vi "temperature_control_1.5.vi"(11 "User":string) -> ()   [LabVIEW 2014]
panel:
  in  "选项卡控件":T1(tab)
  in  "VISA resource name":refnum<visa-resource-name>="COM8" caption="VISA资源名称"
  in  "baud rate (9600)":u32=9600 caption="波特率(9600)"
  in  "data bits (8)":u16=8 caption="数据比特(8)" min=5 max=8 step=1
  in  "parity (0:none)":enum16{"None", "Odd", "Even", "Mark", "Space"}(ring) caption="奇偶（0:无）"
  in  "stop bits (10: 1 bit)":u16(ring)=10 caption="停止位（10: 1位）" items=["1.0"=10, "1.5"=15, "2.0"=20]
  in  "flow control (0:none)":u16(ring) caption="流控制（0:无）" items=["无", "XON/XOFF", "RTS/CTS", "XON/XOFF & RTS/CTS", "DTR/DSR", "XON/XOFF & DTR/DSR"]
  out "Console":string
  out "XY Graph":cluster{"Y":dbl[], "Y":dbl[]}[](graph) caption="XY图"
  out "Hello":string
  in  "Initialization confirm":bool
  in  "Reset":bool
  out "Working Status":string
  in  "电源开关":bool
  in  "变温控制":bool
  in  "停止":bool
  out "变温":bool
  in  "Desitination Value":dbl
  out "Expectation Value":dbl
  out "add_step":dbl=0.008
  in  "变温等待间隙":dbl=1.5 format="%.2f"
  out "电流设置回读":string
  out "电压值回读":string
  out "电压设置回读":string
  out "电流值回读":string
  out "过压设置值回读":string
  out "键盘锁":string="CC"
  out "过压":string="CC"
  out "蜂鸣器":string="CC"
  out "CC/CV":string="CC"
  out "测量模式":string="CC"
  out "过温":string="CC"
  out "On/Off":string="CC"
  out "日期/时间字符串":string
  in  "I-t_data":path
  out "数字":u32
  in  "log":path=path "E:/"
  in  "SET COMMAND":u16(ring) items=["CURRENT SET", "VOLTAGE SET", "ON/OFF", "LOCK SET", "OVPROTECT SET", "SOUND", ""]
  in  "数值":dbl
  in  "SET":bool
  out "RESULT":string
  in  "Read COMMAND":u16(ring) items=["CURRENT SET", "VOLTAGE SET", "ON/OFF", "LOCK SET", "OVPROTECT SET", "SOUND", ""]
  in  "Read":bool
  out "Value":string
  out "log":refnum<file>
  out "I-t data":refnum<file>
  in  "Turning Point4":dbl=4.0
  in  "Turing Pont3":dbl=3.5
  in  "Turning Point2":dbl=2.5
  in  "Turning Point1":dbl=1.5
  in  "step1":dbl=0.01
  in  "step2":dbl=0.008
  in  "step3":dbl=0.006
  in  "step4":dbl=0.005
  in  "step5":dbl=0.004
  in  "精度":dbl=0.01
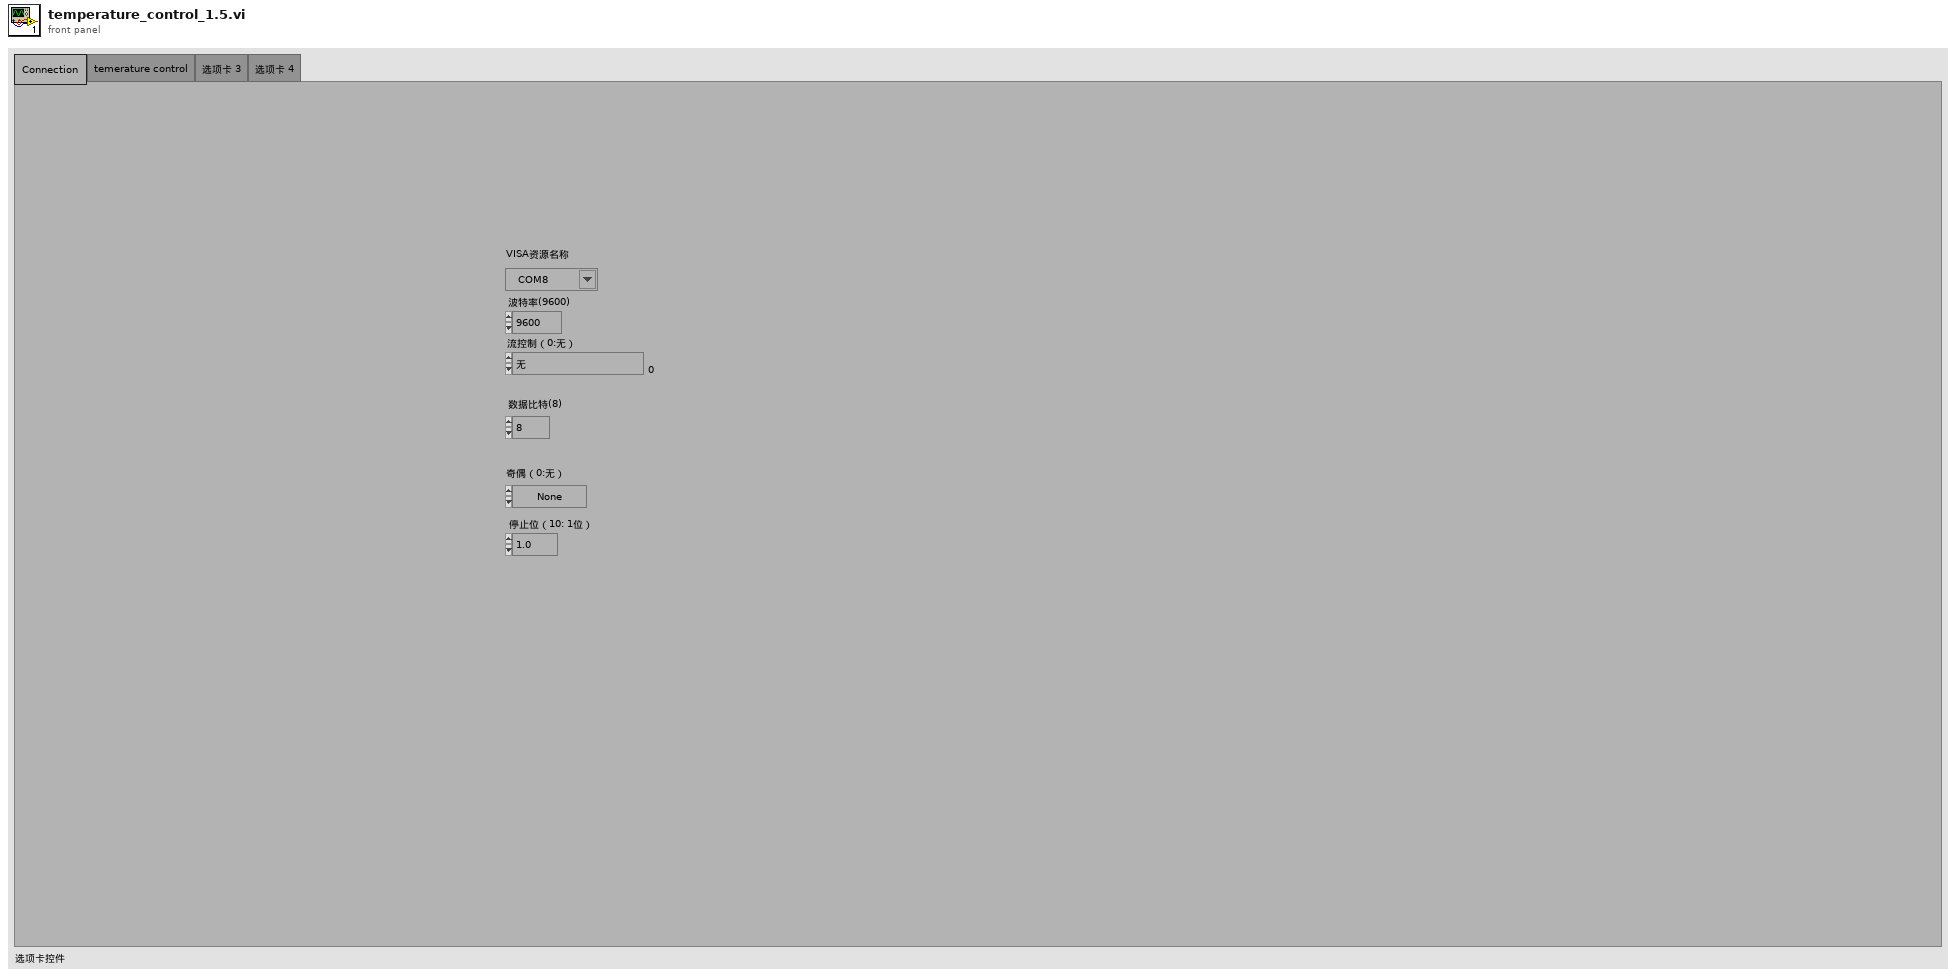
[diagram p1: front panel]
types:
  T1 = enum32{"Connection ", "temerature control", "选项卡 3", "选项卡 4"}
  T2 = enum16{"open", "replace", "create", "open or create", "replace or create", "replace or create with confirmation"}
  T3 = enum8{"Enabled", "Disabled", "Disabled and Grayed Out"}
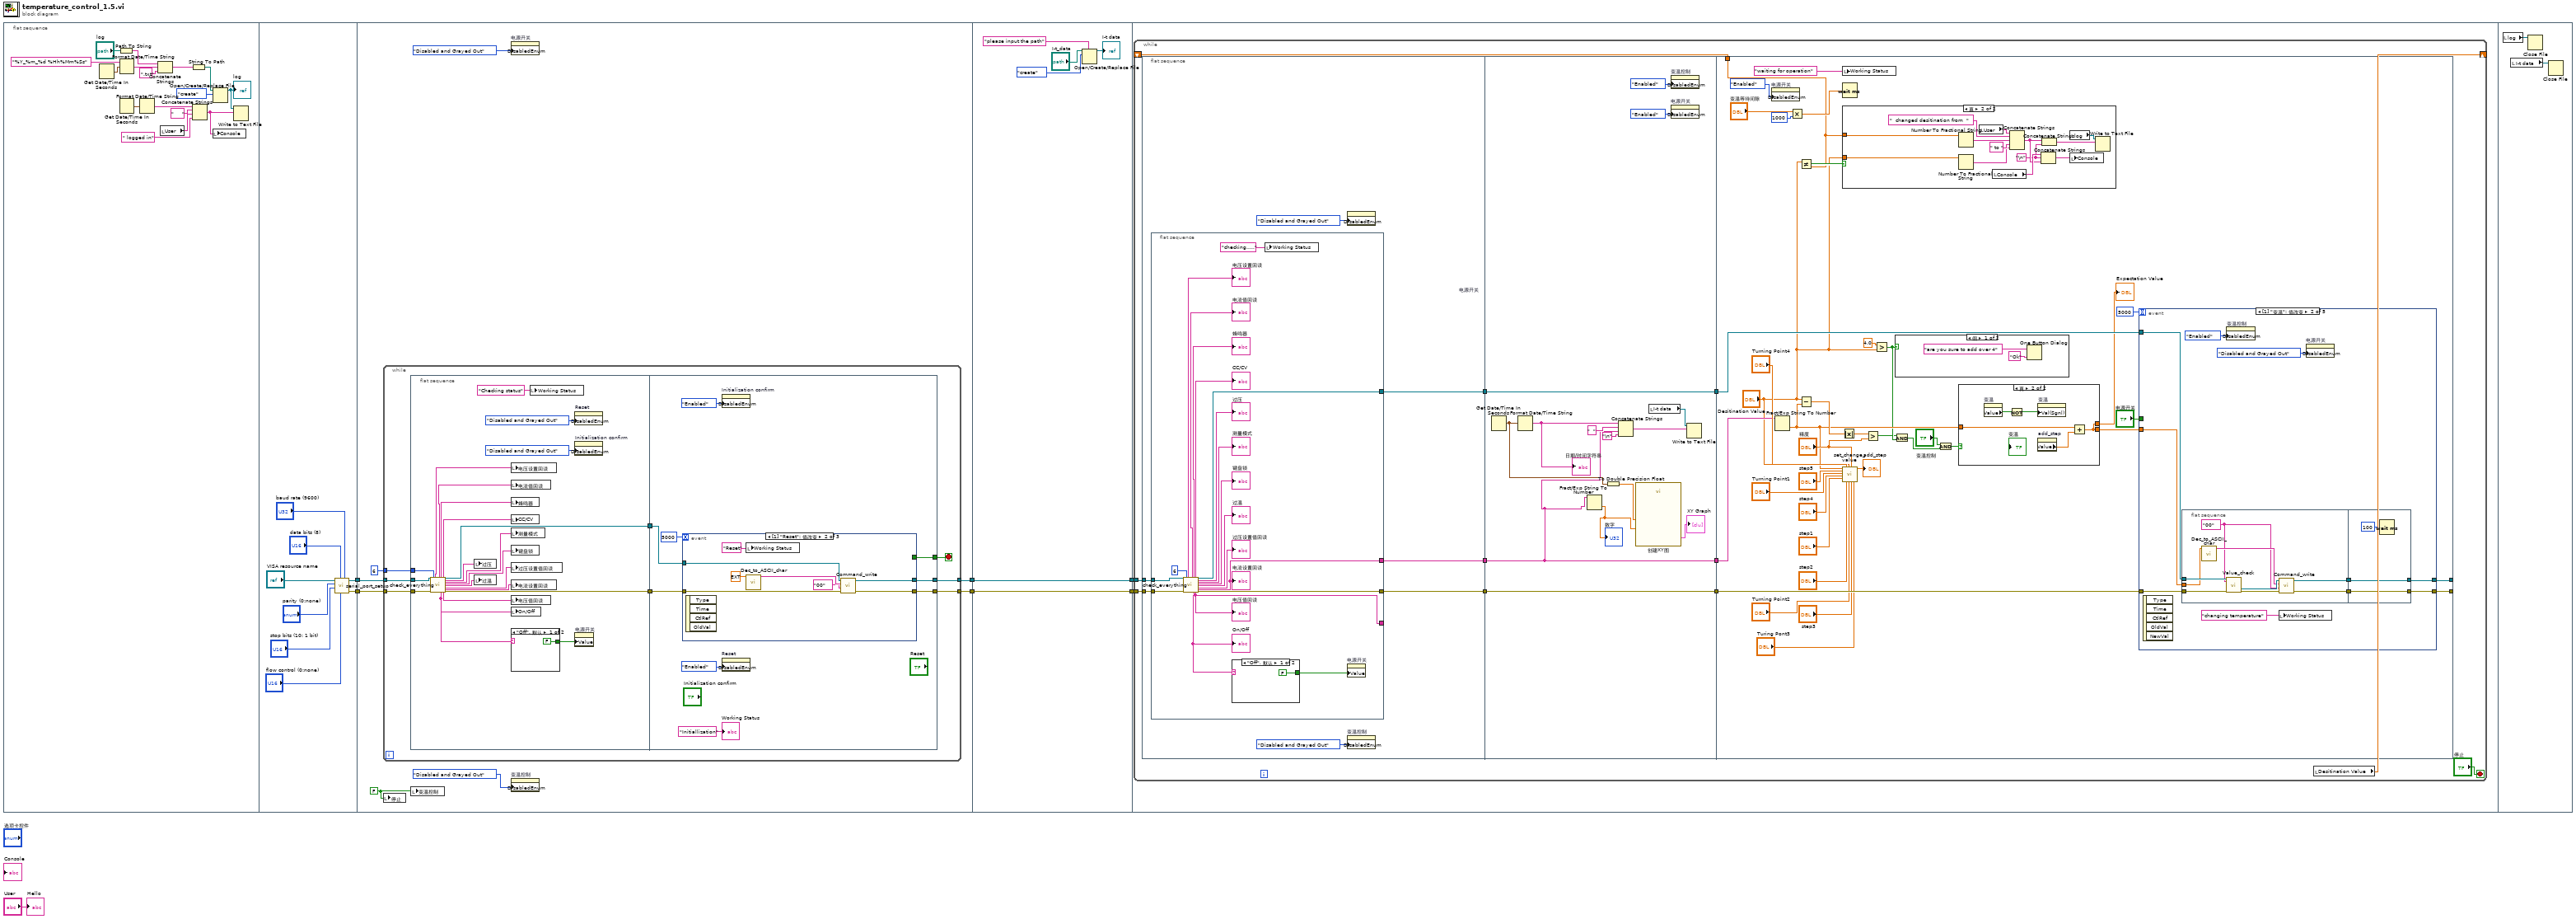
[diagram p0: block diagram]
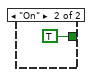
[diagram p2: hidden frame]
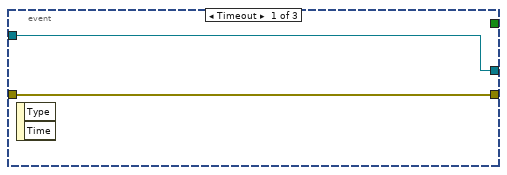
[diagram p3: hidden frame]
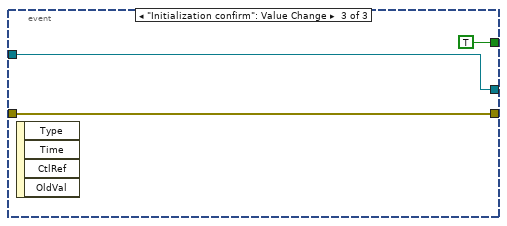
[diagram p4: hidden frame]
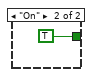
[diagram p5: hidden frame]
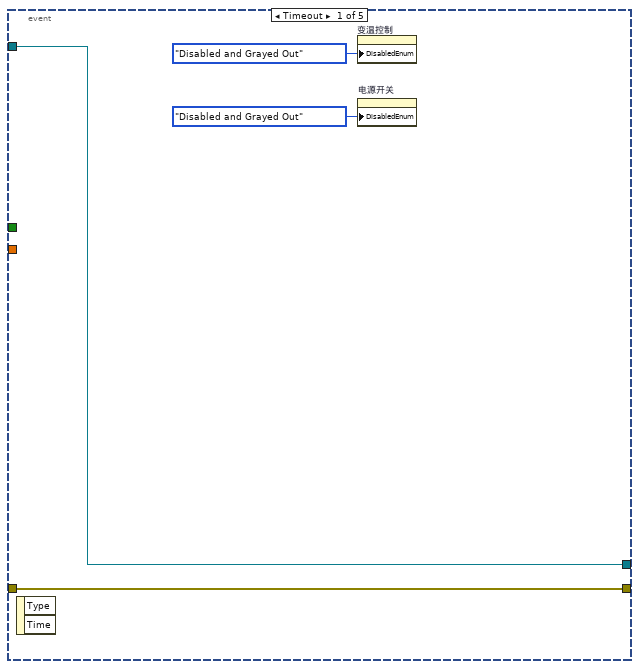
[diagram p9: hidden frame]
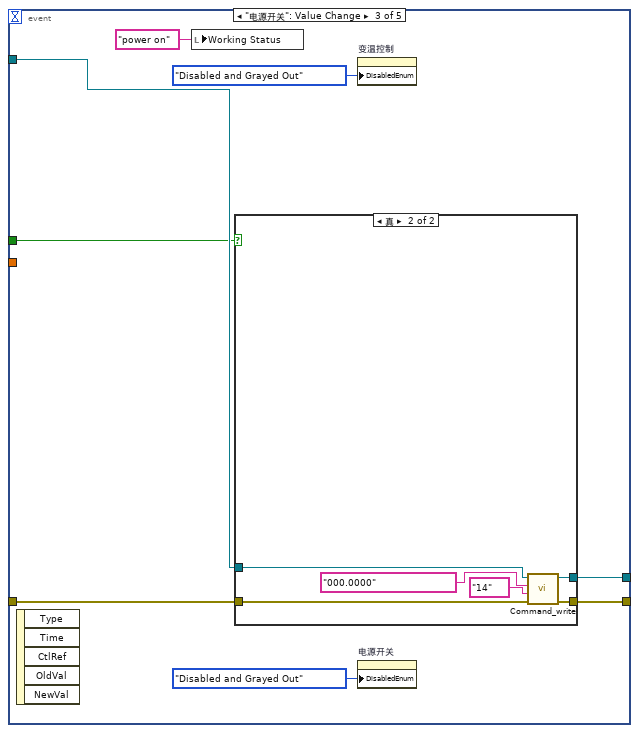
[diagram p10: hidden frame]
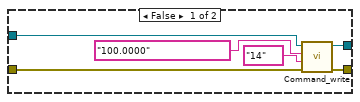
[diagram p11: hidden frame]
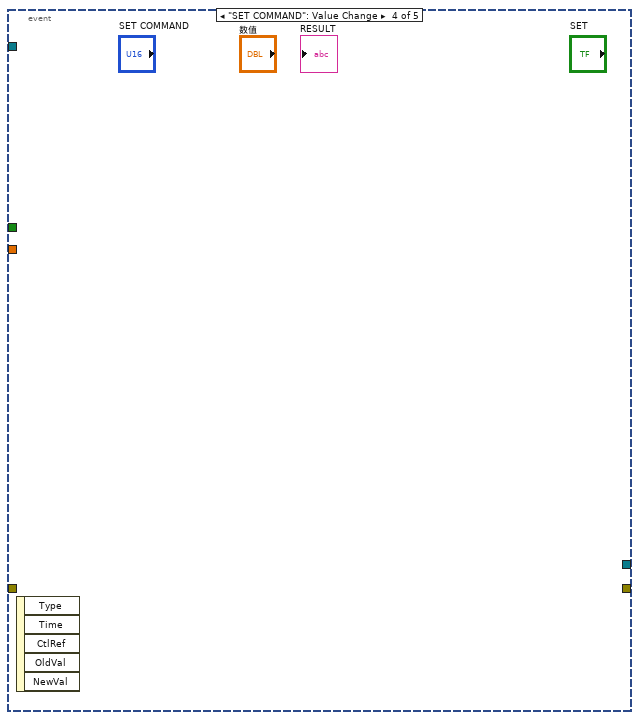
[diagram p12: hidden frame]
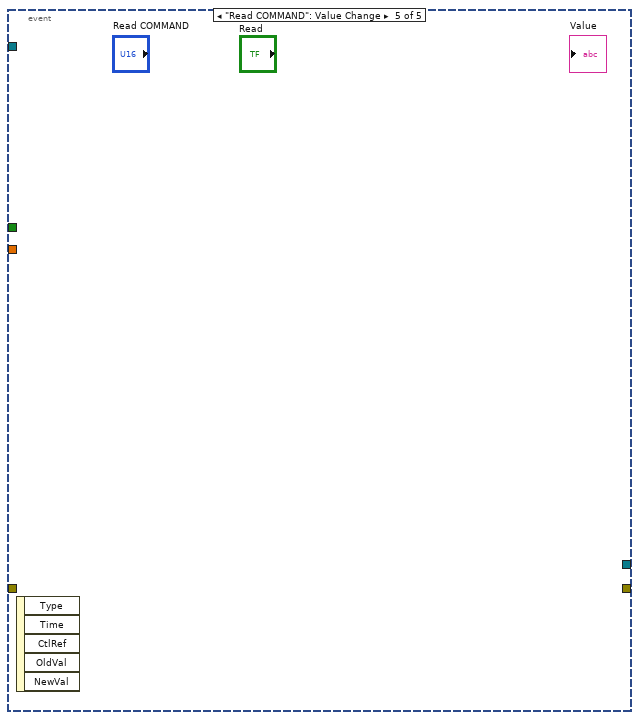
[diagram p13: hidden frame]
diagram:
  n1 = flat-sequence {
    tunnel: [w25] -> w7
    tunnel: [w24] -> w6
    tunnel: [w34] -> w4
    tunnel: w7 -> [w38]
    tunnel: w6 -> [w37]
    tunnel: [w33] -> w2
    tunnel: w4 -> [w98]
    tunnel: [w98] -> w3
    tunnel: w2 -> [w97]
    tunnel: [w97] -> w1
    tunnel: w3 -> [w100]
    tunnel: w1 -> [w99]
    frame #0 {
      n2 = Get Date/Time In Seconds() -> (seconds since 1Jan1904=w12:timestamp)
      n3 = Path To String(path="log") -> (string=w11:string)
      n4 = Format Date/Time String(time format string (%c)="%Y_%m_%d %Hh%Mm%Ss" ("时间格式字符串(%c)"), seconds (now)=w12) -> (date/time string=w17:string)  [unwired: 1 in]
      n5 = Get Date/Time In Seconds() -> (seconds since 1Jan1904=w22:timestamp)
      n6 = Format Date/Time String(seconds (now)=w22) -> (date/time string=w20:string)  [unwired: 2 in]
      n7 = Concatenate Strings(w11, w17, ".txt" ("字符串")) -> (w14:string)
      n8 = local read "User"() -> (w21:string)
      n9 = String To Path(string=w14) -> (path=w15:path)
      n10 = Concatenate Strings(w20, "     " ("字符串"), w21, " logged in" ("Console")) -> (w8:string)
      n11 = Open/Create/Replace File(file path (use dialog)=w15, operation (0:open)=T2."create" ("操作(0:open)")) -> (refnum out=w9:refnum<file>)  [unwired: 4 in, 2 out]
      "log" <- w9
      n12 = local write "Console"(w8) -> ()
      n13 = Write to Text File(file (use dialog)=w9, text=w8) -> ()  [unwired: 2 in, 3 out]
    }
    frame #1 {
      n14 = call "serial_port_setup.vi"("baud rate (9600)"="baud rate (9600)", "flow control (0:none)"="flow control (0:none)", "data bits (8)"="data bits (8)", "stop bits (10: 1 bit)"="stop bits (10: 1 bit)", "parity (0:none)"="parity (0:none)", "VISA引用句柄输入"="VISA resource name") -> ("错误输出"=w24:errorcluster, "VISA引用句柄输出"=w25:refnum<visa-resource-name>)  [unwired: 4 in]
    }
    frame #2 {
      w32 = FALSE ("停止")
      n15 = while {
        tunnel: 6 -> [w47]
        tunnel: w38 -> [w46]
        tunnel: w37 -> [w45]
        tunnel: [w41] -> w34
        tunnel: [w40] -> w33
        stop <- w42 stop-if-true
        n16 = flat-sequence {
          tunnel: w47 -> [w68]
          tunnel: w46 -> [w67]
          tunnel: w45 -> [w66]
          tunnel: [w65] -> w44
          tunnel: [w49] -> w43
          tunnel: w44 -> [w78]
          tunnel: w43 -> [w77]
          tunnel: [w76] -> w42
          tunnel: [w75] -> w41
          tunnel: [w74] -> w40
          frame #0 {
            n17 = call "check_everything.vi"("VISA引用句柄输入"=w67, "错误输入（无错误）"=w66, "数值输入"=w68) -> ("电压设置回读"=w62:string, "电流值回读"=w61:string, "蜂鸣器"=w54:string, "On/Off"=w51:string, "CC/CV"=w60:string, "电压值回读"=w57:string, "VISA引用句柄输出"=w65:refnum<visa-resource-name>, "过压"=w55:string, "测量模式"=w59:string, "键盘锁"=w56:string, "过温"=w58:string, "过压设置值回读"=w53:string, "电流设置回读"=w52:string, "错误输出"=w49:errorcluster)  [unwired: 10 in, 1 out]
            n18 = local write "过压"(w55) -> ()
            n19 = local write "过温"(w58) -> ()
            n20 = local write "电压设置回读"(w62) -> ()
            n21 = local write "电流值回读"(w61) -> ()
            n22 = local write "蜂鸣器"(w54) -> ()
            n23 = local write "CC/CV"(w60) -> ()
            n24 = local write "测量模式"(w59) -> ()
            n25 = local write "键盘锁"(w56) -> ()
            n26 = local write "过压设置值回读"(w53) -> ()
            n27 = local write "电流设置回读"(w52) -> ()
            n28 = local write "电压值回读"(w57) -> ()
            n29 = local write "On/Off"(w51) -> ()
            n30 = case shown="\"Off\", 默认" w51 {
              tunnel: [FALSE TRUE] -> w50
              frame "Off", Default {
              }
              frame "On" {
              }
            }
            n31 = local write "Working Status"("Checking status") -> ()
            n32 = property on="Reset" class="Bool"("DisabledEnum"=T3."Disabled and Grayed Out" ("禁用")) -> ()  [unwired: 2 in, 2 out]
            n33 = property on="Initialization confirm" class="Bool"("DisabledEnum"=T3."Disabled and Grayed Out" ("禁用")) -> ()  [unwired: 2 in, 2 out]
            n34 = property on="电源开关" class="Bool (严格)"("Value"=w50) -> ()  [unwired: 2 in, 2 out]
          }
          frame #1 {
            n35 = event shown="[1] \"Reset\": 值改变" {
              selector: _ -> [_ _ _]
              dyn-events: _ -> [_ _ _]
              timeout: u32 5000 ("y") -> [_ _ _]
              tunnel: [w81 w87 w92] -> w75
              tunnel: w78 -> [w81 w89 w92]
              tunnel: w77 -> [w80 w88 w91]
              tunnel: [w80 w86 w91] -> w74
              tunnel: [_ _ TRUE] -> w76
              event Timeout {
                n36 = event-data() -> ()  [unwired: 1 in, 2 out]
              }
              event "Reset": Value Change {
                n37 = event-data() -> ()  [unwired: 1 in, 4 out]
                n38 = local write "Working Status"("Reset") -> ()
                n39 = call "Dec_to_ASCII_char.vi"("SetPoint"=ext 0.0) -> ("字符串"=w85:string)  [unwired: 10 in]
                n40 = call "Command_write.vi"("错误输入（无错误）"=w88, "Status code"="00", "Data"=w85, "VISA引用句柄输入"=w89) -> ("错误输出"=w86:errorcluster, "VISA引用句柄输出"=w87:refnum<visa-resource-name>)  [unwired: 5 in, 1 out]
              }
              event "Initialization confirm": Value Change {
                n41 = event-data() -> ()  [unwired: 1 in, 4 out]
              }
            }
            n42 = property on="Initialization confirm" class="Bool"("DisabledEnum"=T3."Enabled" ("禁用")) -> ()  [unwired: 2 in, 2 out]
            n43 = property on="Reset" class="Bool"("DisabledEnum"=T3."Enabled" ("禁用")) -> ()  [unwired: 2 in, 2 out]
            "Working Status" <- "Initiallization"
          }
        }
      }
      n44 = local write "停止"(w32) -> ()
      n45 = local write "变温控制"(w32) -> ()
      n46 = property on="电源开关" class="Bool (严格)"("DisabledEnum"=T3."Disabled and Grayed Out" ("禁用")) -> ()  [unwired: 2 in, 2 out]
      n47 = property on="变温控制" class="Bool (严格)"("DisabledEnum"=T3."Disabled and Grayed Out" ("禁用")) -> ()  [unwired: 2 in, 2 out]
    }
    frame #3 {
      n48 = Open/Create/Replace File(file path (use dialog)="I-t_data", prompt="please input the path" ("提示"), operation (0:open)=T2."create" ("操作(0:open)")) -> (refnum out=→"I-t data":refnum<file>)  [unwired: 3 in, 2 out]
    }
    frame #4 {
      n49 = while {
        tunnel: w100 -> [w111]
        tunnel: w99 -> [w110]
        shift-right: [w102] -> _
        shift-left: _ -> [w101]
        stop <- "停止" stop-if-true
        n50 = flat-sequence {
          tunnel: w110 -> [w117]
          tunnel: w111 -> [w118]
          tunnel: [w115] -> w108
          tunnel: [w116] -> w106
          tunnel: [w114] -> w104
          tunnel: w108 -> [w153]
          tunnel: [w153] -> w107
          tunnel: w106 -> [w140]
          tunnel: [w140] -> w105
          tunnel: w104 -> [w152]
          tunnel: [w152] -> w103
          tunnel: [w168] -> _
          tunnel: w107 -> [w189]
          tunnel: w105 -> [w167]
          tunnel: w103 -> [w188]
          tunnel: [w166] -> _
          tunnel: w101 -> [w155]
          frame #0 {
            n51 = flat-sequence {
              tunnel: w118 -> [w127]
              tunnel: w117 -> [w126]
              tunnel: [w125] -> w116
              tunnel: [w124] -> w115
              tunnel: [w123] -> w114
              tunnel: [w119] -> _
              frame #0 {
                n52 = call "check_everything.vi"("VISA引用句柄输入"=w127, "错误输入（无错误）"=w126, "数值输入"=6) -> ("电压设置回读"=→"电压设置回读":string, "电流值回读"=→"电流值回读":string, "蜂鸣器"=→"蜂鸣器":string, "On/Off"=w120:string, "CC/CV"=→"CC/CV":string, "电压值回读"=w119:string, "VISA引用句柄输出"=w124:refnum<visa-resource-name>, "过压"=→"过压":string, "测量模式"=→"测量模式":string, "键盘锁"=→"键盘锁":string, "过温"=→"过温":string, "过压设置值回读"=→"过压设置值回读":string, "电流设置回读"=w125:string, "错误输出"=w123:errorcluster)  [unwired: 10 in, 1 out]
                "On/Off" <- w120
                "电压值回读" <- w119
                "电流设置回读" <- w125
                n53 = case shown="\"Off\", 默认" w120 {
                  tunnel: [FALSE TRUE] -> w121
                  frame "Off", Default {
                  }
                  frame "On" {
                  }
                }
                n54 = local write "Working Status"("checking.....") -> ()
                n55 = property on="电源开关" class="Bool (严格)"("Value"=w121) -> ()  [unwired: 2 in, 2 out]
              }
            }
            n56 = property on="电源开关" class="Bool (严格)"("DisabledEnum"=T3."Disabled and Grayed Out" ("禁用")) -> ()  [unwired: 2 in, 2 out]
            n57 = property on="变温控制" class="Bool (严格)"("DisabledEnum"=T3."Disabled and Grayed Out" ("禁用")) -> ()  [unwired: 2 in, 2 out]
          }
          frame #1 {
            n58 = Get Date/Time In Seconds() -> (seconds since 1Jan1904=w144:timestamp)
            n59 = Format Date/Time String(seconds (now)=w144) -> (date/time string=w145:string)  [unwired: 2 in]
            "日期/时间字符串" <- w145
            n60 = Fract/Exp String To Number(string=w140) -> (number=w141:dbl)  [unwired: 3 in, 1 out]
            "数字" <- w141
            n61 = To Double Precision Float(number=w144) -> (double precision float=w143:dbl)
            n62 = Concatenate Strings(w145, "  " ("字符串"), w140, "\n") -> (w146:string)
            n63 = call "创建XY图"("Y Input"=w141, "X Input"=w143) -> ("XY Graph"=→"XY Graph":cluster{"X":dbl[], "Y":dbl[]}[])  [unwired: 8 in, 1 out]
            n64 = local read "I-t data"() -> (w147:refnum<file>)
            n65 = property on="变温控制" class="Bool (严格)"("DisabledEnum"=T3."Enabled" ("禁用")) -> ()  [unwired: 2 in, 2 out]
            n66 = property on="电源开关" class="Bool (严格)"("DisabledEnum"=T3."Enabled" ("禁用")) -> ()  [unwired: 2 in, 2 out]
            n67 = Write to Text File(file (use dialog)=w147, text=w146) -> ()  [unwired: 2 in, 3 out]
          }
          frame #2 {
            n68 = property on="电源开关" class="Bool (严格)"("DisabledEnum"=T3."Enabled" ("禁用")) -> ()  [unwired: 2 in, 2 out]
            n69 = Fract/Exp String To Number(string=w167) -> (number=w170:dbl)  [unwired: 3 in, 1 out]
            n70 = Multiply(x="变温等待间隙", y=u32 1000) -> (x*y=w164:dbl)
            n71 = Not Equal?(x="Desitination Value", y=w155) -> (x != y?=w156:bool)
            n72 = Subtract(x="Desitination Value", y=w170) -> (x-y=w184:dbl)
            n73 = Absolute Value(x=w184) -> (abs(x)=w183:dbl)
            n74 = local write "Working Status"("waiting for operation") -> ()
            n75 = Wait (ms)(milliseconds to wait=w164) -> ()  [unwired: 1 out]
            n76 = case shown="真" w156 {
              tunnel: w155 -> [_ w194]
              tunnel: "Desitination Value" -> [_ w192]
              frame False {
              }
              frame True {
                w195 = "\n"
                n77 = Number To Fractional String(number=w194) -> (F-format string=w193:string)  [unwired: 3 in]
                n78 = Number To Fractional String(number=w192) -> (F-format string=w191:string)  [unwired: 3 in]
                n79 = local read "User"() -> (w201:string)
                n80 = local read "Console"() -> (w199:string)
                n81 = Concatenate Strings(w201, "  changed desitination from  ", w193, " to " ("字符串"), w191) -> (w196:string)
                n82 = Concatenate Strings(w199, w195, w196) -> (w198:string)
                n83 = Concatenate Strings(w196, w195) -> (w197:string)
                n84 = local read "log"() -> (w203:refnum<file>)
                n85 = local write "Console"(w198) -> ()
                n86 = Write to Text File(file (use dialog)=w203, text=w197) -> ()  [unwired: 2 in, 3 out]
              }
            }
            n87 = call "set_change_value.vi"("数值输入"=w170, "step5"="step5", "Turning Point1"="Turning Point1", "step4"="step4", "step1"="step1", "Turning Point4"="Turning Point4", "step2"="step2", "Desitination Value"="Desitination Value", "Turning Point2"="Turning Point2", "精度"="精度", "step3"="step3", "Turing Pont3"="Turing Pont3") -> ("数值输出"=→"add_step":sgl)  [unwired: 7 in]
            n88 = Greater?(x=w183, y="精度") -> (0:w158:bool)
            n89 = Greater?(x=4.0, y="Desitination Value") -> (0:w159:bool)
            n90 = And(x=w158, y=w159) -> (x .and. y?=w157:bool)
            n91 = case shown="假" w159 {
              frame False {
                n92 = One Button Dialog(message="are you sure to add over 4", button name ("OK")="Ok") -> ()  [unwired: 1 out]
              }
              frame True {
              }
            }
            n93 = And(x="变温控制", y=w157) -> (x .and. y?=w187:bool)
            n94 = case shown="真" w187 {
              tunnel: w170 -> [w206 w209]
              tunnel: [w206 w207] -> w185
              tunnel: [w206 w207] -> w181
              frame False {
              }
              frame True {
                n95 = property on="变温" class="Bool (严格)"() -> ("Value"=w211:bool)  [unwired: 2 in, 2 out]
                n96 = Not(x=w211) -> (.not. x?=w210:bool)
                n97 = property on="变温" class="Bool (严格)"("Val(Sgnl)"=w210) -> ()  [unwired: 2 in, 2 out]
                n98 = property on="add_step" class="DigNum (严格)"() -> ("Value"=w208:dbl)  [unwired: 2 in, 2 out]
                n99 = Add(x=w209, y=w208) -> (x+y=w207:dbl)
              }
            }
            "Expectation Value" <- w181
            n100 = event shown="[1] \"变温\": 值改变" {
              selector: _ -> [_ _ _ _ _]
              dyn-events: _ -> [_ _ _ _ _]
              timeout: 5000 -> [_ _ _ _ _]
              tunnel: w189 -> [w215 w225 w245 _ _]
              tunnel: w188 -> [w214 w224 w244 _ _]
              tunnel: [w215 w223 w243 _ _] -> w168
              tunnel: [w214 w222 w242 _ _] -> w166
              tunnel: w185 -> [_ w221 _ _ _]
              tunnel: "电源开关" -> [_ _ w241 _ _]
              event Timeout {
                n101 = event-data() -> ()  [unwired: 1 in, 2 out]
                n102 = property on="变温控制" class="Bool (严格)"("DisabledEnum"=T3."Disabled and Grayed Out" ("禁用")) -> ()  [unwired: 2 in, 2 out]
                n103 = property on="电源开关" class="Bool (严格)"("DisabledEnum"=T3."Disabled and Grayed Out" ("禁用")) -> ()  [unwired: 2 in, 2 out]
              }
              event "变温": Value Change {
                n104 = event-data() -> ()  [unwired: 1 in, 5 out]
                n105 = flat-sequence {
                  tunnel: w225 -> [w232]
                  tunnel: w224 -> [w231]
                  tunnel: w221 -> [w228]
                  tunnel: [w230] -> w219
                  tunnel: [w229] -> w218
                  tunnel: [w236] -> w222
                  tunnel: [w237] -> w223
                  tunnel: w219 -> [w237]
                  tunnel: w218 -> [w236]
                  frame #0 {
                    w226 = "00"
                    n106 = call "Dec_to_ASCII_char.vi"("SetPoint"=w228) -> ("字符串"=w227:string)  [unwired: 10 in]
                    n107 = call "Value_check.vi"("VISA引用句柄输入"=w232, "Status Code"=w226, "错误输入（无错误）"=w231) -> ("VISA资源名称输出"=w234:refnum<visa-resource-name>, "错误输出"=w233:errorcluster)  [unwired: 3 in, 12 out]
                    n108 = call "Command_write.vi"("错误输入（无错误）"=w233, "Status code"=w226, "Data"=w227, "VISA引用句柄输入"=w234) -> ("错误输出"=w229:errorcluster, "VISA引用句柄输出"=w230:refnum<visa-resource-name>)  [unwired: 5 in, 1 out]
                  }
                  frame #1 {
                    n109 = Wait (ms)(milliseconds to wait=u32 100 ("等待时间（毫秒）")) -> ()  [unwired: 1 out]
                  }
                }
                n110 = property on="变温控制" class="Bool (严格)"("DisabledEnum"=T3."Enabled" ("禁用")) -> ()  [unwired: 2 in, 2 out]
                n111 = local write "Working Status"("changing temperature") -> ()
                n112 = property on="电源开关" class="Bool (严格)"("DisabledEnum"=T3."Disabled and Grayed Out" ("禁用")) -> ()  [unwired: 2 in, 2 out]
              }
              event "电源开关": Value Change {
                n113 = event-data() -> ()  [unwired: 1 in, 5 out]
                n114 = local write "Working Status"("power on" ("Working Status")) -> ()
                n115 = case shown="真" w241 {
                  tunnel: w245 -> [w249 w257]
                  tunnel: w244 -> [w248 w256]
                  tunnel: [w247 w255] -> w243
                  tunnel: [w246 w254] -> w242
                  frame False {
                    n116 = call "Command_write.vi"("错误输入（无错误）"=w248, "Status code"="14", "Data"="100.0000", "VISA引用句柄输入"=w249) -> ("错误输出"=w246:errorcluster, "VISA引用句柄输出"=w247:refnum<visa-resource-name>)  [unwired: 5 in, 1 out]
                  }
                  frame True {
                    n117 = call "Command_write.vi"("错误输入（无错误）"=w256, "Status code"="14", "Data"="000.0000", "VISA引用句柄输入"=w257) -> ("错误输出"=w254:errorcluster, "VISA引用句柄输出"=w255:refnum<visa-resource-name>)  [unwired: 5 in, 1 out]
                  }
                }
                n118 = property on="变温控制" class="Bool (严格)"("DisabledEnum"=T3."Disabled and Grayed Out" ("禁用")) -> ()  [unwired: 2 in, 2 out]
                n119 = property on="电源开关" class="Bool (严格)"("DisabledEnum"=T3."Disabled and Grayed Out" ("禁用")) -> ()  [unwired: 2 in, 2 out]
              }
              event "SET COMMAND": Value Change {
                n120 = event-data() -> ()  [unwired: 1 in, 5 out]
              }
              event "Read COMMAND": Value Change {
                n121 = event-data() -> ()  [unwired: 1 in, 5 out]
              }
            }
          }
        }
        n122 = local read "Desitination Value"() -> (w102:dbl)
      }
    }
    frame #5 {
      n123 = local read "log"() -> (w258:refnum<file>)
      n124 = local read "I-t data"() -> (w259:refnum<file>)
      n125 = Close File(refnum=w258) -> ()  [unwired: 1 in, 2 out]
      n126 = Close File(refnum=w259) -> ()  [unwired: 1 in, 2 out]
    }
  }
  "Hello" <- "User"
